vi "JLT_Query.vi"(0 "System no.":i32=1 min=1 max=4 step=1, 1 "Joystick IDs":i32[](array[numeric]), 2 "Joystick axes":i32[](array[numeric]), 3 "Without parameter?":bool, 5 "error in":errorcluster, 6 "Xo":i32=1, 7 "N":i32=100) -> (14 "Data":dbl[][](array[numeric]) format="%.2f", 15 "Names":string[](array[string]), 16 "JLT? string":string, 19 "error out":errorcluster)   [LabVIEW 2020]
doc: "Returns joystick lookup table for joysticks connected to the controller. For large N values, communication timeout must be set long enough, otherwise a comm.error may occur.\n\nC-867, E-709, E-861, E-870, Mercury_GCS: JoystickIDs and Joystick axes must be omitted in the JLT? command, while X0 and N are always required.\n\nE-709: Only supported if E-709 is used inside C-867K012/K013."
uses:
  whitespace.ctl
panel:
  # "Returns joystick lookup table for joysticks connected to the controller. For large N values, communication \ntimeout must be set long enough, otherwise a comm.error may occur."
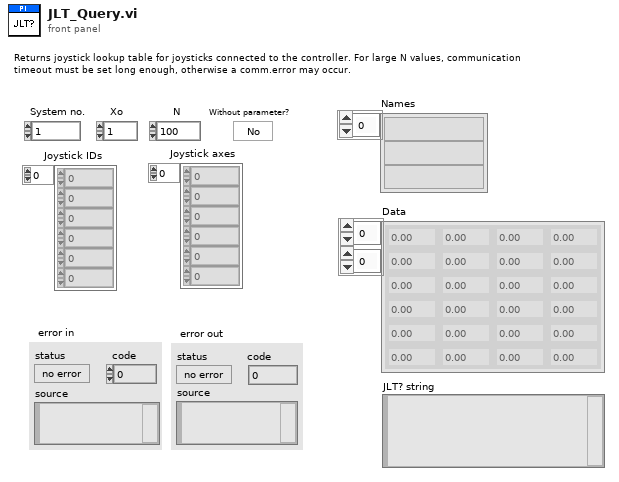
[diagram p1: front panel]
types:
  T1 = cluster{"Read (F)/Write":bool, "Path":path, "Datastream":string, "ArrayName":string}
  T2 = typedef "whitespace.ctl" = u16
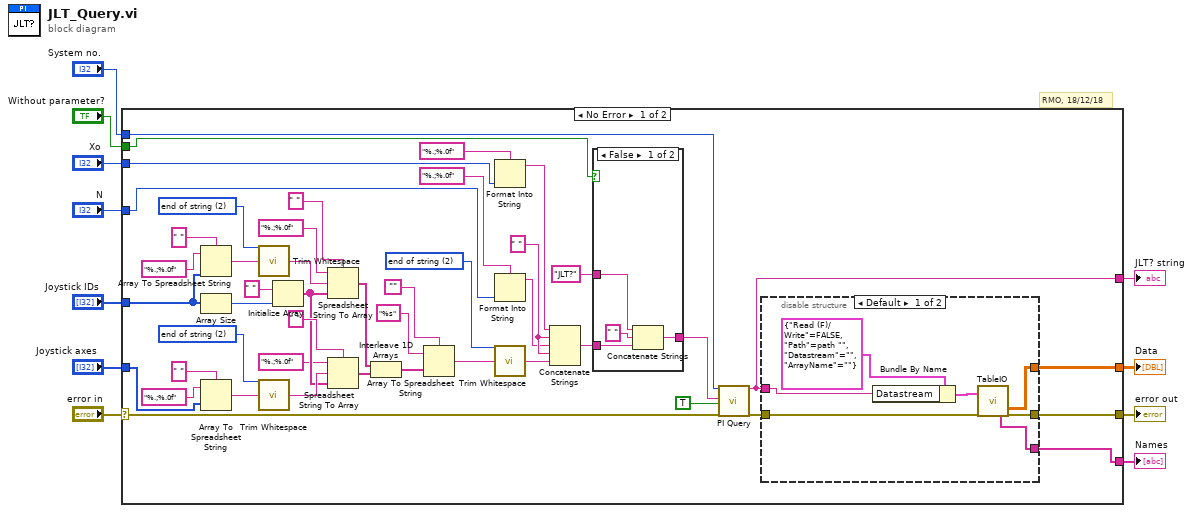
[diagram p0: block diagram]
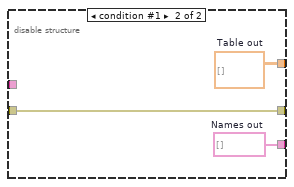
[diagram p2: hidden frame]
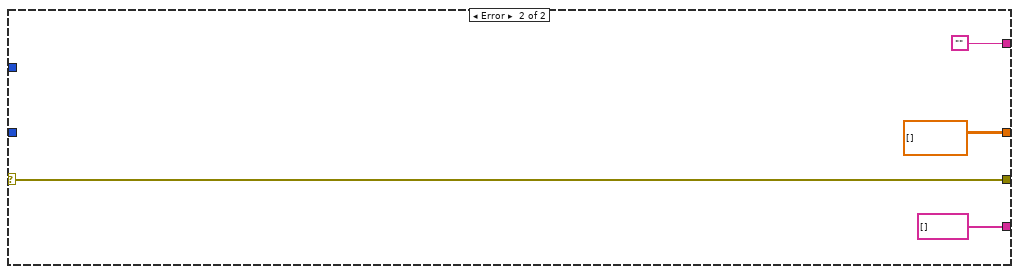
[diagram p4: hidden frame]
diagram:
  # "RMO, 18/12/18"
  n1 = case shown="No Error" "error in" {
    selector: "error in" -> [w14 w73]
    tunnel: "System no." -> [w55 _]
    tunnel: "Joystick IDs" -> [w32 _]
    tunnel: [w53 w73] -> w10
    tunnel: [w52 dbl[][] [] ("Table out")] -> w7
    tunnel: "N" -> [w48 _]
    tunnel: "Xo" -> [w50 _]
    tunnel: [w47 string[] [] ("Names out")] -> w6
    tunnel: "Without parameter?" -> [w41 _]
    tunnel: "Joystick axes" -> [w37 _]
    tunnel: [w12 ""] -> w2
    frame No Error {
      w21 = T2 2 items=["both", "start of string", "end of string"] ("location (both)")
      w34 = T2 2 items=["both", "start of string", "end of string"] ("location (both)")
      w35 = T2 2 items=["both", "start of string", "end of string"] ("location (both)")
      w49 = " "
      n2 = Array To Spreadsheet String(delimiter (Tab)=" ", array=w32, 3:"%.;%.0f" ("Format String")) -> (spreadsheet string=w36:string)
      n3 = Array Size(array=w32) -> (size(s)=w31:i32)
      n4 = Array To Spreadsheet String(delimiter (Tab)=" ", array=w37, 3:"%.;%.0f" ("Format String")) -> (spreadsheet string=w33:string)
      n5 = call "Trim Whitespace.vi"("string"=w36, "location (both)"=w35) -> ("trimmed string"=w29:string)
      n6 = call "Trim Whitespace.vi"("string"=w33, "location (both)"=w34) -> ("trimmed string"=w28:string)
      n7 = Initialize Array(" ", w31) -> (w24:string[])
      n8 = Spreadsheet String To Array(delimiter (Tab)=" ", format string="%.;%.0f" ("Format String"), spreadsheet string=w29, array type (2D Dbl)=w24) -> (array=w25:string[])
      n9 = Spreadsheet String To Array(delimiter (Tab)=" ", format string="%.;%.0f" ("Format String"), spreadsheet string=w28, array type (2D Dbl)=w24) -> (array=w23:string[])
      n10 = Interleave 1D Arrays(w25, w23) -> (w22:string[])
      n11 = Array To Spreadsheet String(delimiter (Tab)="", array=w22, 3:"%s" ("Format String")) -> (spreadsheet string=w20:string)
      n12 = Format Into String(format string="%.;%.0f" ("Format String"), w50) -> (resulting string=w46:string)  [unwired: 2 in, 1 out]
      n13 = Format Into String(format string="%.;%.0f" ("Format String"), w48) -> (resulting string=w45:string)  [unwired: 2 in, 1 out]
      n14 = call "Trim Whitespace.vi"("string"=w20, "location (both)"=w21) -> ("trimmed string"=w19:string)
      n15 = Concatenate Strings(w46, w49, w45, w49, w19) -> (w42:string)
      n16 = case shown="False" w41 {
        tunnel: "JLT?" -> [w71 w72]
        tunnel: [w70 w72] -> w56
        tunnel: w42 -> [w69 _]
        frame False {
          n17 = Concatenate Strings(w71, " " ("Substring"), w69) -> (w70:string)
        }
        frame True {
        }
      }
      n18 = call "PI Query.vi"("System no."=w55, "String to send"=w56, "Attach termination char.?"=TRUE ("Attach Linefeed?"), "error in"=w14) -> ("String read"=w12:string, "error out"=w13:errorcluster)  [unwired: 3 in, 11 out]
      n19 = disable-structure shown="Default" {
        disable-tunnel: [w64 w67] -> w53
        disable-tunnel: [w63 w65] -> w52
        disable-tunnel: [w61 w66] -> w47
        disable-tunnel: w13 -> [w59 w67]
        disable-tunnel: w12 -> [w58 _]
        frame condition #0 (active) {
          n20 = Bundle By Name(cluster=T1 {"Read (F)/Write"=FALSE, "Path"=path "", "Datastream"="", "ArrayName"=""} ("IOSource"), "Datastream"=w58) -> (w60:T1)
          n21 = call "TableIO.vi"("IOSource"=w60, "error in"=w59) -> ("Names out"=w61:string[], "Table out"=w63:dbl[][], "error out"=w64:errorcluster)  [unwired: 4 in, 11 out]
        }
        frame condition #1 {
          w65 = dbl[][] []  # Table out
          w66 = string[] []  # Names out
        }
      }
    }
    frame Error {
    }
  }
  "error out" <- w10
  "Data" <- w7
  "Names" <- w6
  "JLT? string" <- w2
